vi "Global - Monitoring Variables.vi"() -> ()   [LabVIEW 2020]
uses:
  controls/FPGA VI Reference.ctl
panel:
  in  "Send Live Data":bool
  in  "Live Data Channel":u32
  in  "Drive Space":dbl
  in  "Current FPGA VI Reference":T1
  in  "Buffer Backlog":dbl
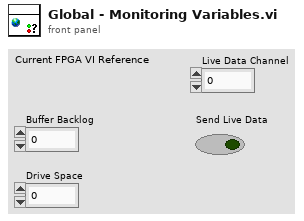
[diagram p1: front panel]
types:
  T1 = typedef "FPGA VI Reference.ctl" = refnum<k20>
diagram:
